vi "LHF.DB.Mongo.Util.GetDocumentPart.vi"(6 "Extract _id (T)":bool=TRUE, 7 "projection type":variant, 8 "error in (no error)":errorcluster, 9 "_id":string, 10 "Collection":string, 11 "LHF.DB.Mongo in":refnum<class "LHF.DB.Mongo.lvclass">) -> (0 "error out":errorcluster, 1 "_id":string, 2 "Document":variant, 3 "LHF.DB.Mongo out":refnum<class "LHF.DB.Mongo.lvclass">)   [LabVIEW 2013, in "LHF.DB.Mongo.lvclass"]
uses:
  LHF.DB.Mongo.lvclass
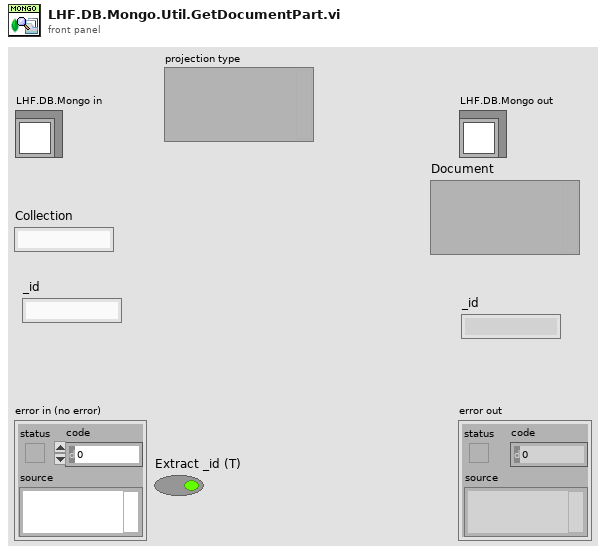
[diagram p1: front panel]
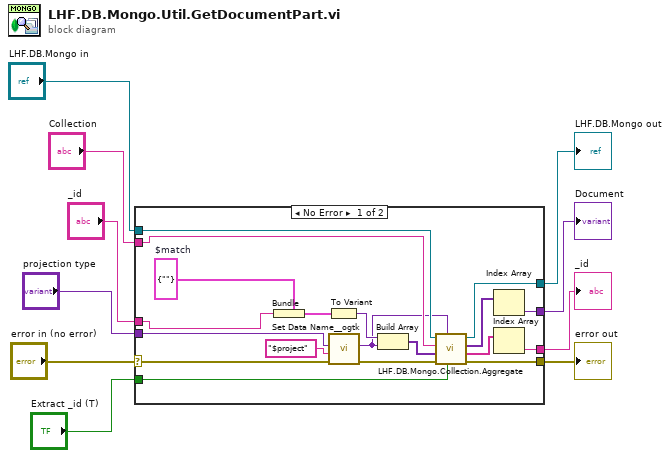
[diagram p0: block diagram]
diagram:
  n1 = case shown="No Error" "error in (no error)" {
    selector: "error in (no error)" -> [w13 w31]
    tunnel: [w21 w31] -> w9
    tunnel: [w28 w30] -> w7
    tunnel: "LHF.DB.Mongo in" -> [w27 w30]
    tunnel: "Collection" -> [w29 _]
    tunnel: [w25 _] -> w5
    tunnel: "projection type" -> [w19 _]
    tunnel: "_id" -> [w17 _]
    tunnel: [w23 _] -> w2
    tunnel: "Extract _id (T)" -> [w22 _]
    frame No Error {
      w18 = cluster{"_id":string} {"_id"=""}  # $match
      n2 = Bundle(cluster=w18, "_id"=w17) -> (w16:cluster{"_id":string})
      n3 = To Variant(anything=w16) -> (Variant=w15:variant)
      n4 = call <userlib>:"Set Data Name__ogtk.vi"("error in (no error)"=w13, "Data Name"="$project", "Data"=w19) -> ("error out"=w12:errorcluster, "Renamed Data"=w11:variant)  [unwired: 7 in]
      n5 = Build Array(w15, w11) -> (w14:variant[])
      n6 = call-dynamic "LHF.DB.Mongo.Collection.Aggregate.vi"("Extract _id (T)"=w22, "return type"=w11, "error in (no error)"=w12, "Operations"=w14, "Collection"=w29, "LHF.DB.Mongo in"=w27) -> ("error out"=w21:errorcluster, "_id Array"=w24:string[], "Documents"=w26:variant[], "LHF.DB.Mongo out"=w28:refnum<class "LHF.DB.Mongo.lvclass">)  [unwired: 2 in]
      n7 = Index Array(array=w26) -> (element=w25:variant)  [unwired: 1 in]
      n8 = Index Array(array=w24) -> (element=w23:string)  [unwired: 1 in]
    }
    frame Error {
    }
  }
  "error out" <- w9
  "LHF.DB.Mongo out" <- w7
  "Document" <- w5
  "_id" <- w2
